vi "ManualTrigger.vi"() -> ()   [LabVIEW 2016]
uses:
  <vilib>/Platform/TimedLoop/XDataNode/timing_clust.ctl
  <vilib>/Platform/TimedLoop/XDataNode/nitl_modes.ctl
  <vilib>/Platform/TimedLoop/XDataNode/wakeup.ctl
  <vilib>/DAQmx/write.llb/DAQmx Write (Digital Bool 1Line 1Point).vi
  <vilib>/DAQmx/create/channels.llb/DAQmx Create Channel (DO-Digital Output).vi
  <vilib>/DAQmx/miscellaneous.llb/DAQmx Fill In Error Info.vi
  <vilib>/platform/TimedLoop/XDataNode/XDataNode.xnode
  <vilib>/Platform/TimedLoop/XDataNode/XDNodeRunTimeDep.lvlib
panel:
  out "Cycles":i32
  in  "Toggle":bool
  in  "High":u32=250
  in  "Low":i64=3000
  in  "Mode":enum32{"Continuous pulse", "Manual Switch"}(radio)
  out "error out":errorcluster
  out "Display":bool
  in  "stop":bool
  in  "error in":errorcluster
  # "Pulse (us)"
  # "Manual"
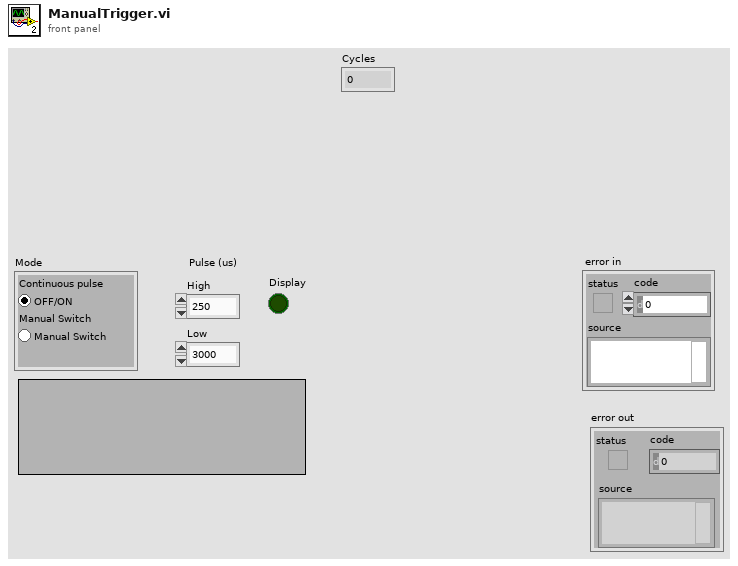
[diagram p1: front panel]
types:
  T1 = typedef "XDNodeRunTimeDep.lvlib/timing_clust.ctl" = cluster{"Expected End [f-1]":u64, "Actual End [f-1]":u64, "Finished Late? [f-1]":bool, "Expected End [i-1]":u64, "Actual End [i-1]":u64, "Finished Late? [i-1]":bool, "Expected Start [i]":u64, "Actual Start [i]":u64, "Expected Start [f]":u64, "Actual Start [f]":u64, "Source Name":string, "Structure Name":string, "Period":i64, "Deadline":i64, "Offset":i64, "Start":i64, "Priority":i32, "Timeout":i32, "Mode":T2, "Wakeup Reason":T3, "Error":errorcluster, "Source Type":string, "Secondary Source Type":string, "Global End Time":u64, "Global Start Time":u64, "Frame Duration":u64, "Iteration Duration":u64, "Assigned CPU":i32, "I/O Scan Engine Mode":u32}
  T2 = typedef "XDNodeRunTimeDep.lvlib/nitl_modes.ctl" = enum32{"No Change", "Process missed periods, maintain original phase", "Discard missed periods, maintain original phase", "Process missed periods, ignore original phase", "Discard missed periods, ignore original phase"}
  T3 = typedef "XDNodeRunTimeDep.lvlib/wakeup.ctl" = enum32{"Normal", "Aborted", "Asynchronous wakeup", "Timing source error", "Timed loop error", "Timeout"}
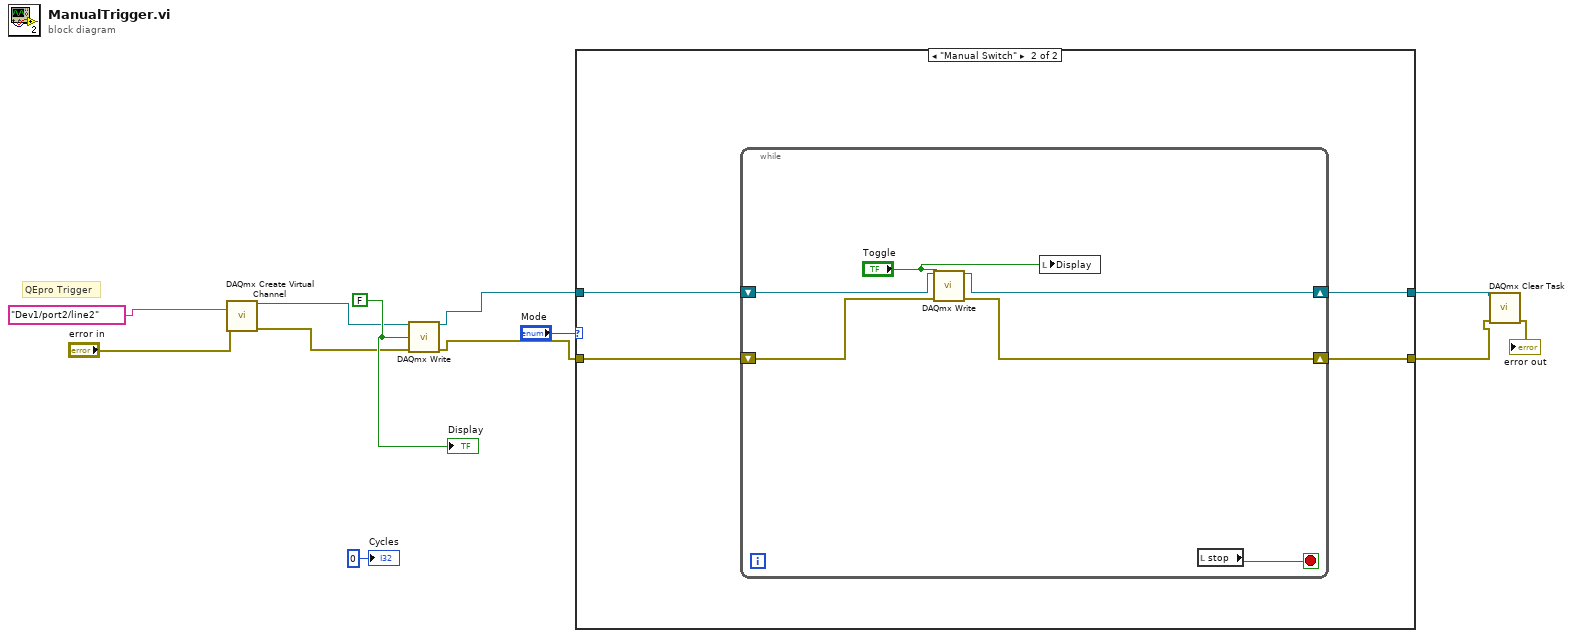
[diagram p0: block diagram]
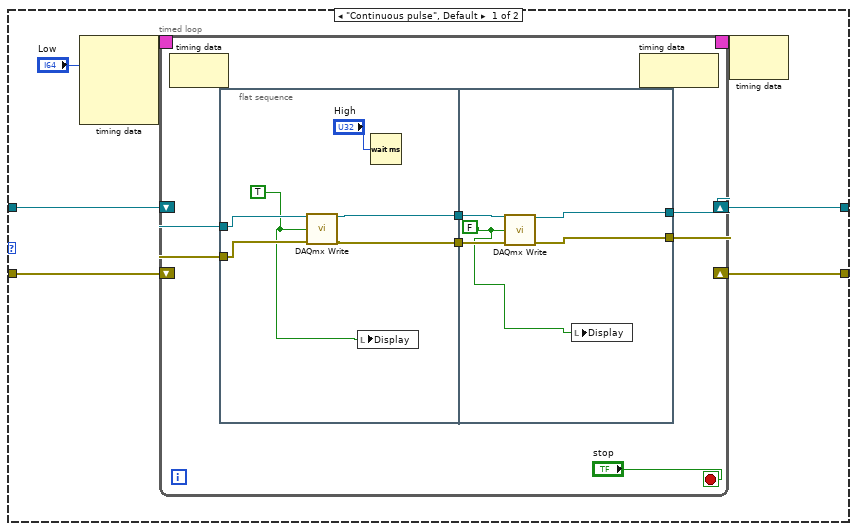
[diagram p2: hidden frame]
diagram:
  w12 = FALSE ("State 2")
  # "QEpro Trigger"
  n1 = call-poly <vilib>:"DAQmx Create Virtual Channel.vi"("lines"=tag "Dev1/port2/line2", "error in"="error in") -> ("task out"=w8:refnum<k21>, "error out"=w9:errorcluster)  [unwired: 12 in]
  n2 = call-poly <vilib>:"DAQmx Write.vi"("task/channels in"=w8, "data"=w12, "error in"=w9) -> ("task out"=w4:refnum<k21>, "error out"=w5:errorcluster)  [unwired: 10 in, 1 out]
  n3 = case shown="\"Manual Switch\"" "Mode" {
    tunnel: [w16 w44] -> w6
    tunnel: w5 -> [w15 w46]
    tunnel: w4 -> [w14 w47]
    tunnel: [w13 w45] -> w3
    frame "Continuous pulse", Default {
      n4 = node-c288("Low") -> (w19:T1)  [unwired: 3 in]
      n5 = timed-loop {
        timing: w19 -> [_]
        timing-out: [_] -> w18
        shift-right: [w23] -> w16
        shift-left: w14 -> [w20]
        shift-right: [w22] -> w13
        shift-left: w15 -> [w21]
        stop <- "stop" stop-if-true
        n6 = node-c288() -> ()  [unwired: 1 in, 1 out]
        n7 = flat-sequence {
          tunnel: [w33] -> w25
          tunnel: [w32] -> w24
          tunnel: w21 -> [w31]
          tunnel: w20 -> [w30]
          tunnel: w25 -> [w39]
          tunnel: w24 -> [w38]
          tunnel: [w36] -> w23
          tunnel: [w35] -> w22
          frame #0 {
            w29 = TRUE ("State 2")
            n8 = call-poly <vilib>:"DAQmx Write.vi"("task/channels in"=w30, "data"=w29, "error in"=w31) -> ("task out"=w33:refnum<k21>, "error out"=w32:errorcluster)  [unwired: 10 in, 1 out]
            n9 = local write "Display"(w29) -> ()
            n10 = Wait (ms)(milliseconds to wait="High") -> ()  [unwired: 1 out]
          }
          frame #1 {
            w37 = FALSE ("State")
            n11 = call-poly <vilib>:"DAQmx Write.vi"("task/channels in"=w39, "data"=w37, "error in"=w38) -> ("task out"=w36:refnum<k21>, "error out"=w35:errorcluster)  [unwired: 10 in, 1 out]
            n12 = local write "Display"(w37) -> ()
          }
        }
        n13 = node-c288() -> ()  [unwired: 1 in, 1 out]
      }
      n14 = node-c288(w18) -> ()  [unwired: 1 out]
    }
    frame "Manual Switch" {
      n15 = while {
        shift-right: [w49] -> w44
        shift-left: w47 -> [w53]
        shift-right: [w51] -> w45
        shift-left: w46 -> [w52]
        stop <- w50 stop-if-true
        n16 = call-poly <vilib>:"DAQmx Write.vi"("task/channels in"=w53, "data"="Toggle", "error in"=w52) -> ("task out"=w49:refnum<k21>, "error out"=w51:errorcluster)  [unwired: 10 in, 1 out]
        n17 = local write "Display"("Toggle") -> ()
        n18 = local read "stop"() -> (w50:bool)
      }
    }
  }
  n19 = call <vilib>:"DAQmx Clear Task.vi"("task in"=w6, "error in"=w3) -> ("error out"=→"error out":errorcluster)  [unwired: 13 in]
  "Display" <- w12
  "Cycles" <- 0 ("Cycles")
